vi "Build VIPB Spec.vi"() -> ()   [LabVIEW 2014]
doc: "This VI will execute a VIPM build\n\nArguments:\nVIPB file path\nBuild number"
uses:
  <userlib>/_OpenG.lib/file/file.llb/Convert File Extension (Path)__ogtk.vi
  <vilib>/Wiresmith Technology/LabVIEW CLI/CLI Class/CLI.lvclass
  <vilib>/JKI/VIPM API/VIPM API_vipm_api.lvlib
panel:
  out "error out":errorcluster
  out "Build Output":path
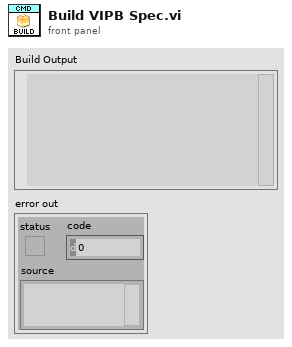
[diagram p1: front panel]
types:
  T1 = typedef "VIPM API_vipm_api.lvlib/VI Package Build Spec Data Cluster_vipm_api.ctl" = cluster{"Package Version":T2, "Product Name":string, "Company Name":string, "Author Name (Person or Company)":string, "Product Homepage (URL)":string, "Legal Copyright":string, "License Agreement Name":string, "Product Description Summary":string, "Product Description":string, "Release Notes - Change Log":string}
  T2 = typedef "VIPM API_vipm_api.lvlib/Version Info Cluster_vipm_api.ctl" = cluster{"major":u32, "minor":u32, "patch":u32, "build":u32}
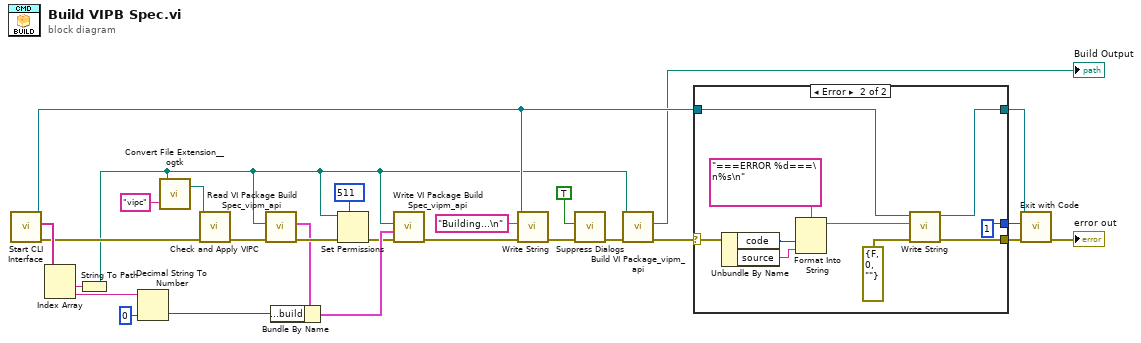
[diagram p0: block diagram]
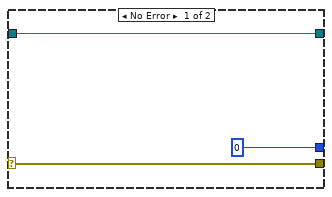
[diagram p2: hidden frame]
diagram:
  n1 = call <vilib>:"Start CLI Interface.vi"() -> ("error out"=w2:errorcluster, "Custom Parameters"=w24:string[], "CLI out"=w21:refnum<class "CLI.lvclass">)  [unwired: 9 in]
  n2 = Index Array(array=w24) -> (element #1=w26:string, element #2=w6:string)  [unwired: 2 in]
  n3 = String To Path(string=w26) -> (path=w1:path)
  n4 = Decimal String To Number(string=w6, default (0L)=u32 0 ("Package Version.build")) -> (number=w25:u32)  [unwired: 1 in, 1 out]
  n5 = call-poly <userlib>:"Convert File Extension__ogtk.vi"("new ending (none)"="vipc", "file name"=w1) -> ("new filename"=w4:path)  [unwired: 1 out]
  n6 = call "Check and Apply VIPC.vi"("error in (no error)"=w2, "VIPC File Path"=w4) -> ("error out"=w3:errorcluster)  [unwired: 9 in]
  n7 = call <vilib>:"Read VI Package Build Spec_vipm_api.vi"("error in (no error)"=w3, "Path to VIPB File"=w1) -> ("error out"=w15:errorcluster, "VI Package Build Spec Data"=w9:T1)  [unwired: 8 in]
  n8 = Bundle By Name(cluster=w9, "Package Version.build"=w25) -> (w17:T1)
  n9 = Set Permissions(7:i16 511 ("permissions"), 8:w15, 11:w1) -> (0:w14:errorcluster)  [unwired: 2 in, 1 out]
  n10 = call <vilib>:"Write VI Package Build Spec_vipm_api.vi"("error in (no error)"=w14, "VI Package Build Spec Data"=w17, "Path to VIPB File"=w1) -> ("error out"=w23:errorcluster)  [unwired: 8 in]
  n11 = call <vilib>:"Write String.vi"("error in (no error)"=w23, "Text to Write"="Building...\n", "CLI in"=w21) -> ("error out"=w12:errorcluster)  [unwired: 7 in, 1 out]
  n12 = call "Suppress Dialogs.vi"("error in (no error)"=w12, "Suppress Dialogs? (F)"=TRUE) -> ("error out"=w11:errorcluster)  [unwired: 9 in]
  n13 = call <vilib>:"Build VI Package_vipm_api.vi"("error in (no error)"=w11, "Path to VIPB File"=w1) -> ("error out"=w7:errorcluster, "Build Output"=→"Build Output":path)  [unwired: 8 in]
  n14 = case shown="Error" w7 {
    selector: w7 -> [w30 w37]
    tunnel: w21 -> [w29 w33]
    tunnel: [w30 w36] -> w20
    tunnel: [w29 w35] -> w18
    tunnel: [0 1] -> w19
    frame No Error {
    }
    frame Error {
      n15 = Unbundle By Name(w37) -> ("code"=w38:i32, "source"=w40:string)
      n16 = Format Into String(format string="===ERROR %d===\n%s\n", w38, w40) -> (resulting string=w31:string)  [unwired: 2 in, 1 out]
      n17 = call <vilib>:"Write String.vi"("error in (no error)"=errorcluster {"status"=FALSE, "code"=0, "source"=""} ("error out"), "Text to Write"=w31, "CLI in"=w33) -> ("error out"=w36:errorcluster, "CLI out"=w35:refnum<class "CLI.lvclass">)  [unwired: 7 in]
    }
  }
  n18 = call <vilib>:"Exit with Code.vi"("error in (no error)"=w20, "Exit Code (0)"=w19, "CLI in"=w18) -> ("error out"=→"error out":errorcluster)  [unwired: 8 in]
